vi "DataBaseConnected.vi"(7 "Get/Set":T2, 11 "BD in":T1 items=["Server", "Local DB"]) -> (3 "BD out":T1 items=["Server", "Local DB"])   [LabVIEW 2019]
uses:
  TypeDef/#TypeDef_DBMode.ctl
  Communication/TypeDef/#TypeDef_SetGet.ctl
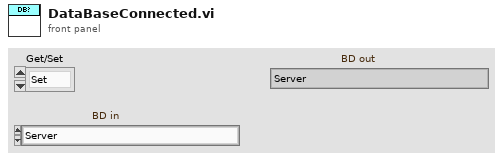
[diagram p1: front panel]
types:
  T1 = typedef "#TypeDef_DBMode.ctl" = u16
  T2 = typedef "#TypeDef_SetGet.ctl" = enum16{"Set", "Get"}
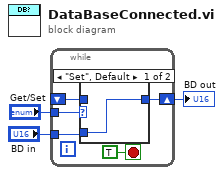
[diagram p0: block diagram]
diagram:
  n1 = while {
    shift-right: [w7] -> w1
    shift-left: _ -> [w5]
    tunnel: "Get/Set" -> [w6]
    tunnel: "BD in" -> [w4]
    stop <- TRUE stop-if-true
    n2 = case shown="\"Set\", Default" w6 {
      tunnel: w5 -> [_ w10]
      tunnel: w4 -> [w9 _]
      tunnel: [w9 w10] -> w7
      frame "Set", Default {
      }
      frame "Get" {
      }
    }
  }
  "BD out" <- w1
